vi "NI VeriStand - Get Channel Block Data References.vi"(8 "error in (no error)":errorcluster, 9 "Access":T4, 10 "Channel Refs":T1[](array[typedef]) format="%.0x", 11 "Device Ref in":T1=18446744073709551615 format="%.0x") -> (0 "error out":errorcluster, 1 "Values Array":dbl[](array[numeric]), 2 "Block Data Refs":T2[](array[typedef]) {"Data Reference" format="%.0x"}, 3 "Device Ref out":T1=18446744073709551615 format="%.0x")   [LabVIEW 2020, in "Custom Device API.lvlib"]
doc: "Returns an array of 32-bit data references to the inline custom device channels specified by <B>Channel Refs</B>. This VI also returns the channel values. You can use the <B>Block Data Refs</B> with the Get Channel Values by Block Data Reference and Set Channel Values by Block Data Reference VIs."
uses:
  <vilib>/NI VeriStand/Custom Device API/Custom Device API.lvlib
  <vilib>/NI VeriStand/Custom Device API/Custom Device Item Ref.ctl
  <vilib>/NI VeriStand/Custom Device API/Data Access Type.ctl
  <vilib>/NI VeriStand/Custom Device API/Block Data Reference.ctl
  <vilib>/NI VeriStand/Custom Device API/Data Reference.ctl
  3b180b88-933f-42ba-a671-11c9dceeb83c.vi
  <vilib>/NI VeriStand/Custom Device API/Custom Device Offline Path.vi
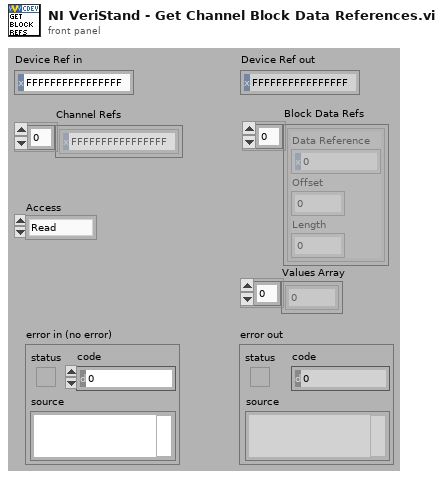
[diagram p1: front panel]
types:
  T1 = typedef "Custom Device API.lvlib/Custom Device Item Ref.ctl" = u64
  T2 = typedef "Custom Device API.lvlib/Block Data Reference.ctl" = cluster{"Data Reference":T3, "Offset":u64, "Length":u64}
  T3 = typedef "Custom Device API.lvlib/Data Reference.ctl" = i32
  T4 = typedef "Custom Device API.lvlib/Data Access Type.ctl" = enum16{"Read", "Write"}
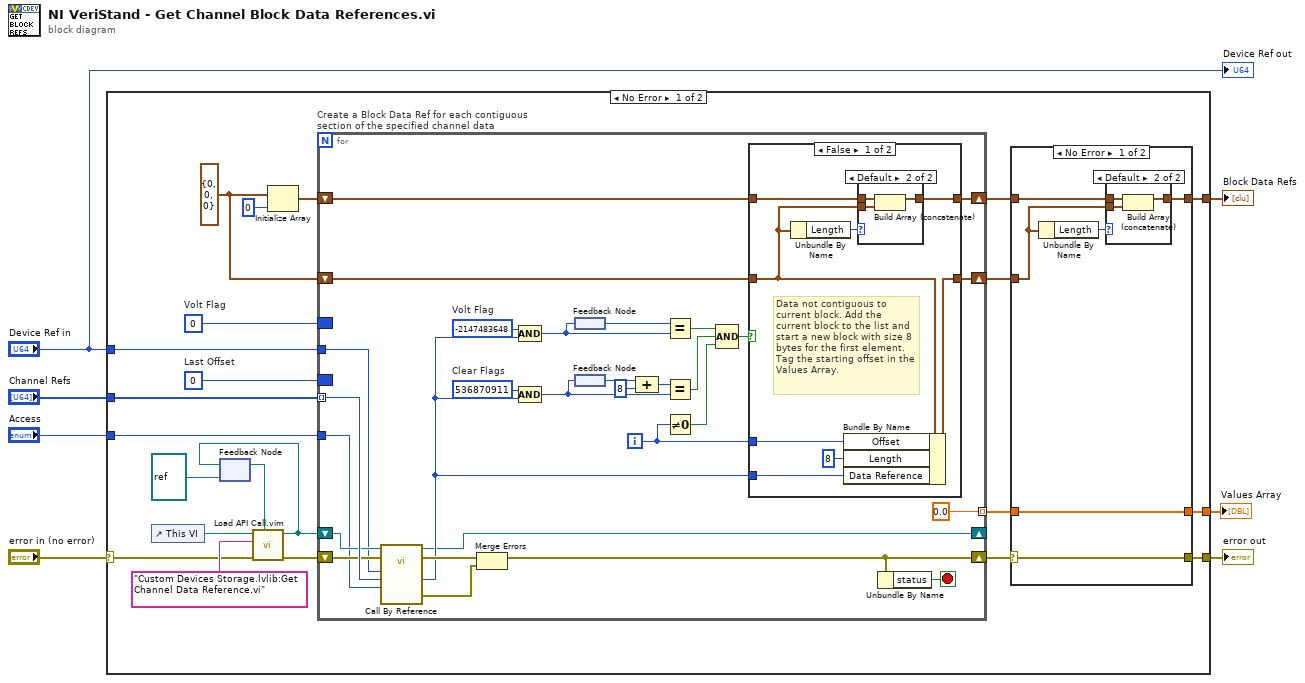
[diagram p0: block diagram]
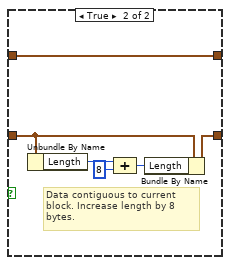
[diagram p3: hidden frame]
diagram:
  n1 = case shown="No Error" "error in (no error)" {
    selector: "error in (no error)" -> [w8 w88]
    tunnel: [w18 w88] -> w7
    tunnel: "Access" -> [w29 _]
    tunnel: "Channel Refs" -> [w28 _]
    tunnel: "Device Ref in" -> [w21 _]
    tunnel: [w23 _] -> w4
    tunnel: [w17 _] -> w1
    frame No Error {
      w25 = T2 {"Data Reference"=0, "Offset"=0, "Length"=0} ("Block Data Ref")
      w19 = 0  # Last Offset
      w20 = 0  # Volt Flag
      n2 = control-ref of="This VI"() -> (w14:refnum<vi>)
      n3 = feedback #1(refnum<vi> refnum ("type specifier VI Refnum (for type only)")) -> (w15:refnum<vi>)
      n4 = call "Load API Call.vim"("VI reference in"=w15, "error in (no error)"=w8, "VI qualified name"="Custom Devices Storage.lvlib:Get Channel Data Reference.vi", "Caller VI ref"=w14) -> ("error out"=w12:errorcluster, "VI reference"=w13:refnum<vi>)  [unwired: 6 in]
      n5 = feedback-in #1(w13) -> ()
      n6 = Initialize Array(w25, 0 ("dimension size")) -> (w26:T2[])
      n7 = for "Create a Block Data Ref for each contiguous section of the specified channel data" {
        shift-right: [w31] -> w9
        shift-left: w12 -> [w38]
        tunnel: w29 -> [w33]
        tunnel: w28 -> [w58] mode=indexing
        shift-right: [w47] -> w24
        shift-left: w26 -> [w48]
        border: w19 -> [_]
        shift-right: [w49] -> w22
        shift-left: w25 -> [w57]
        tunnel: w21 -> [w35]
        tunnel: [0.0 ("element")] -> w16 mode=indexing
        border: w20 -> [_]
        shift-right: [w32] -> _
        shift-left: w13 -> [w36]
        i -> [w41]
        stop <- w39 stop-if-true
        w55 = 536870911  # Clear Flags
        w56 = -2147483648  # Volt Flag
        n8 = call-by-ref "?"(reference=w36, error in=w38, "Access"=w33, "Channel Ref in"=w58, "Device Ref in"=w35) -> (reference out=w32:refnum<vi>, error out=w37:errorcluster, 0:"error out"=w30:errorcluster, "Channel Data Reference"=w34:T3)  [unwired: 6 in, 1 out]
        n9 = Merge Errors(w37, w30) -> (w31:errorcluster)
        n10 = Compound Arithmetic op=AND(w56, w34) -> (w42:T3)
        n11 = Compound Arithmetic op=AND(w55, w34) -> (w52:T3)
        n12 = feedback-in #2(w42) -> ()
        n13 = feedback #2() -> (w43:T3)
        n14 = feedback-in #3(w52) -> ()
        n15 = feedback #3() -> (w53:T3)
        n16 = Compound Arithmetic op=ADD(w53, T3 8 ("value")) -> (w54:T3)
        n17 = Equal?(x=w43, y=w42) -> (x = y?=w45:bool)
        n18 = Equal?(x=w54, y=w52) -> (x = y?=w50:bool)
        n19 = Not Equal To 0?(x=w41) -> (x != 0?=w40:bool)
        n20 = Compound Arithmetic op=AND(w45, w50, w40) -> (w46:bool)
        n21 = case shown="False" w46 {
          tunnel: w57 -> [w63 w76]
          tunnel: [w60 w73] -> w49
          tunnel: w48 -> [w65 w72]
          tunnel: [w64 w72] -> w47
          tunnel: w34 -> [w62 _]
          tunnel: w41 -> [w59 _]
          frame False {
            # "Data not contiguous to current block. Add the current block to the list and start a new block with size 8 bytes for the first element. Tag the starting offset in the Values Array."
            n22 = Unbundle By Name(w63) -> ("Length"=w66:u64)
            n23 = Bundle By Name(cluster=w63, "Offset"=w59, "Length"=u64 8, "Data Reference"=w62) -> (w60:T2)
            n24 = case shown="Default" w66 {
              tunnel: w65 -> [w67 w70]
              tunnel: w63 -> [_ w69]
              tunnel: [w67 w68] -> w64
              frame 0 {
              }
              frame Default {
                n25 = Build Array (concatenate)(w70, w69) -> (w68:T2[])
              }
            }
          }
          frame True {
            # "Data contiguous to current block. Increase length by 8 bytes."
            n26 = Unbundle By Name(w76) -> ("Length"=w75:u64)
            n27 = Compound Arithmetic op=ADD(w75, u64 8 ("value")) -> (w74:u64)
            n28 = Bundle By Name(cluster=w76, "Length"=w74) -> (w73:T2)
          }
        }
        n29 = Unbundle By Name(w31) -> ("status"=w39:bool)
      }
      n30 = case shown="No Error" w9 {
        selector: w9 -> [w78 w87]
        tunnel: w24 -> [w81 _]
        tunnel: [w80 _] -> w23
        tunnel: w22 -> [w79 _]
        tunnel: [w78 w87] -> w18
        tunnel: [w77 _] -> w17
        tunnel: w16 -> [w77 _]
        frame No Error {
          n31 = Unbundle By Name(w79) -> ("Length"=w82:u64)
          n32 = case shown="Default" w82 {
            tunnel: w81 -> [w83 w86]
            tunnel: w79 -> [_ w85]
            tunnel: [w83 w84] -> w80
            frame 0 {
            }
            frame Default {
              n33 = Build Array (concatenate)(w86, w85) -> (w84:T2[])
            }
          }
        }
        frame Error {
        }
      }
    }
    frame Error {
    }
  }
  "error out" <- w7
  "Block Data Refs" <- w4
  "Values Array" <- w1
  "Device Ref out" <- "Device Ref in"
